vi "SeCrTS-DD NS Receiver Storage.vi"(8 "error in":errorcluster) -> ()   [LabVIEW 2022 SP3]
uses:
  Control/SeCrTS-Notifier Ref.ctl
  Globals/SeCrTS-DD globals.vi
  <resource>/objmgr/ni.dex.rc
panel:
  out "x":u32
  out "error out":errorcluster
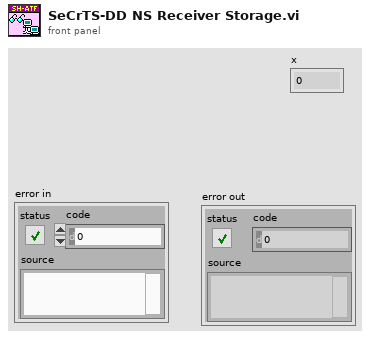
[diagram p1: front panel]
types:
  T1 = typedef "SeCrTS-Notifier Ref.ctl" = cluster{"Pump":refnum<notifier>, "Storage":refnum<notifier>}
  T2 = cluster{"In Progress":bool, "reader url":refnum<k21>, "DI P\nDI S":refnum<queue>[], "analog queue":refnum<queue>[], "NOT DIS Out":T1}
  T3 = enum16{"Initialize", "Wait for connection", "Send data", "Exit", "Receive Data"}
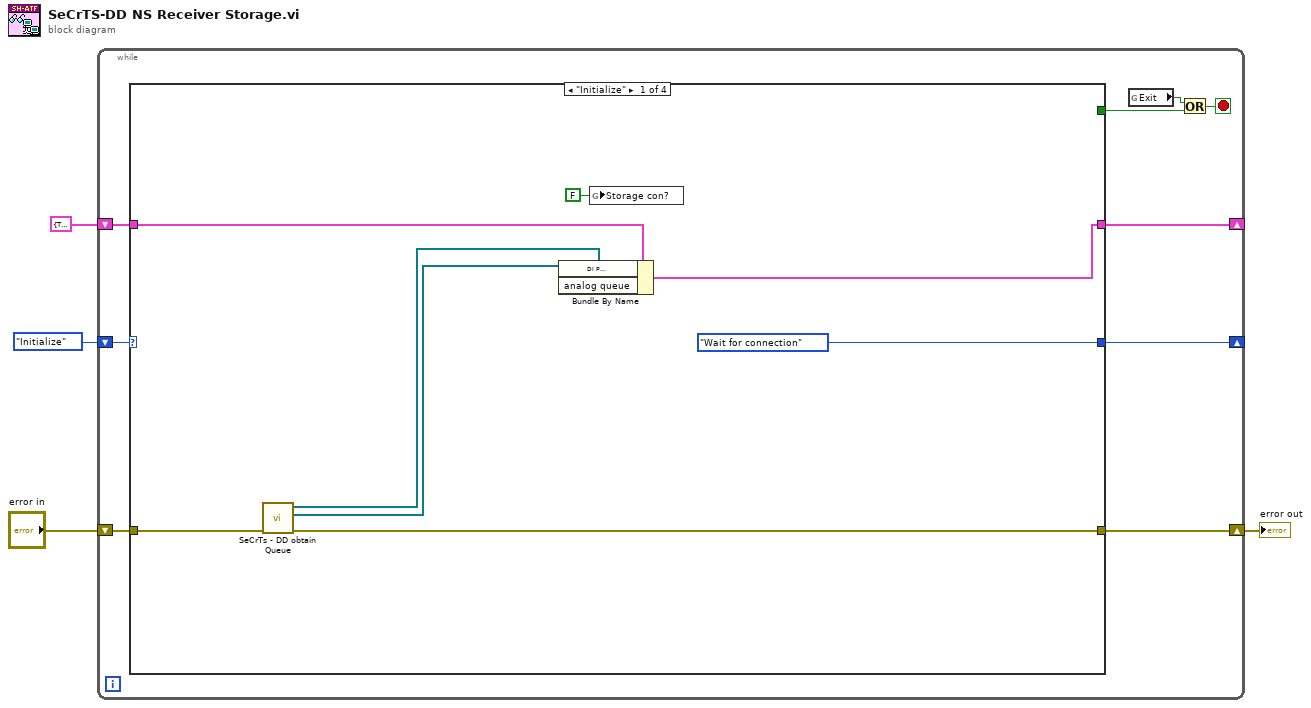
[diagram p0: block diagram]
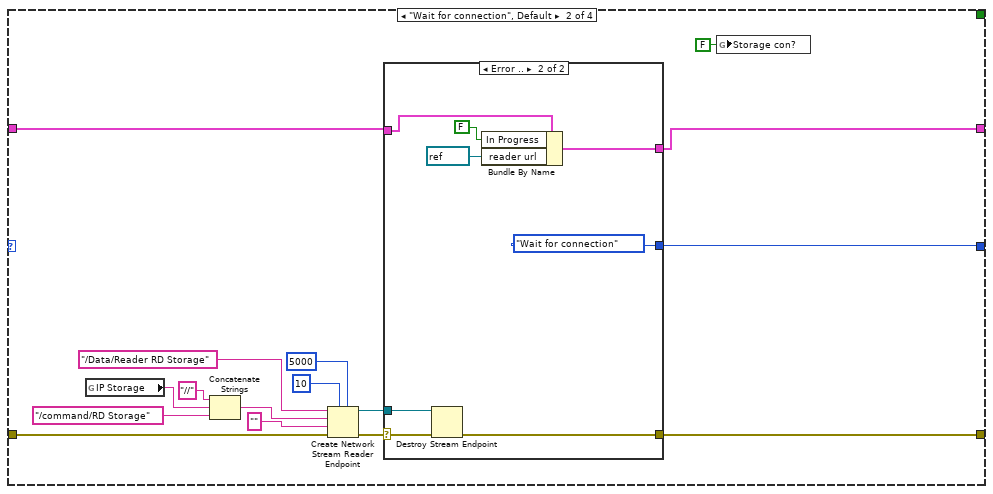
[diagram p2: hidden frame]
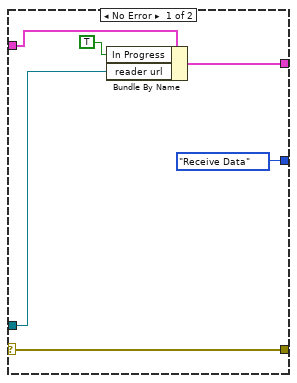
[diagram p3: hidden frame]
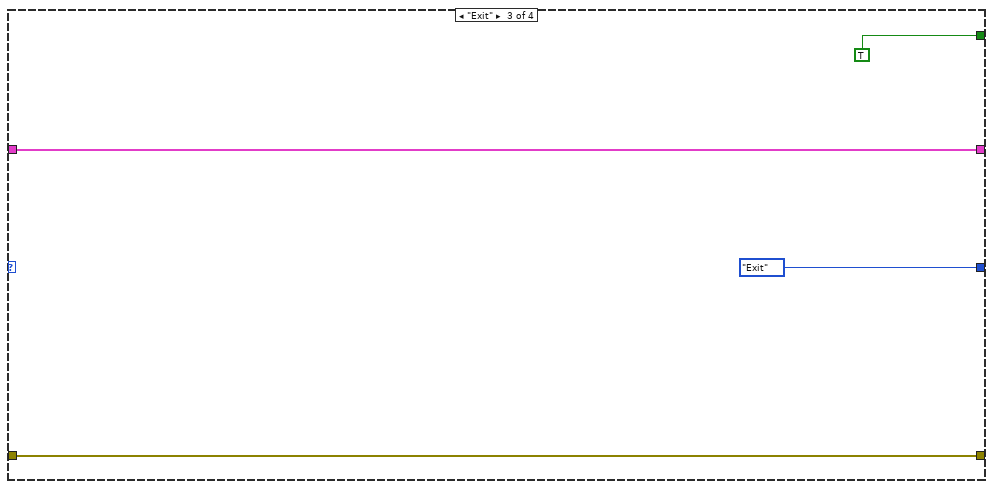
[diagram p4: hidden frame]
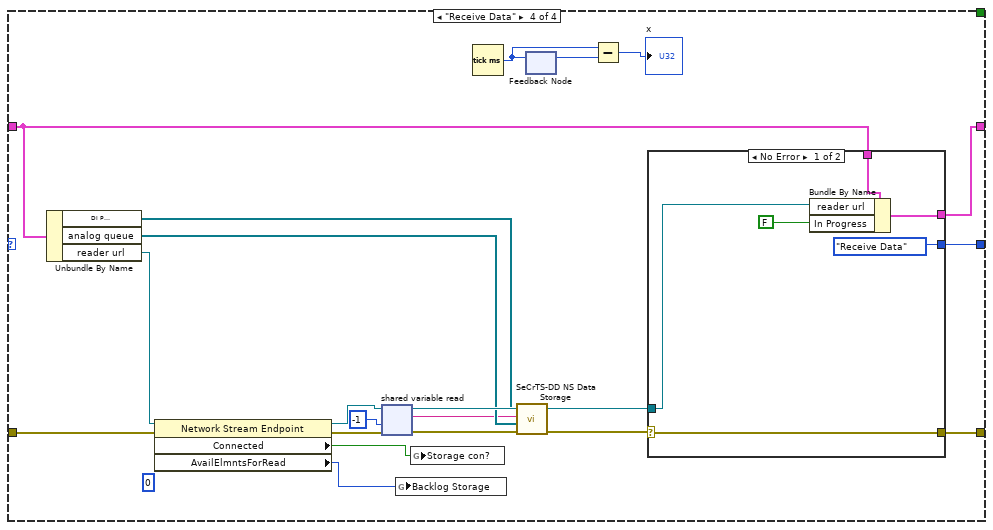
[diagram p5: hidden frame]
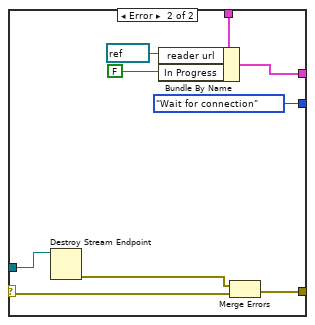
[diagram p6: hidden frame]
diagram:
  n1 = while {
    shift-right: [w11] -> _
    shift-left: T3."Initialize" -> [w13]
    shift-right: [w9] -> _
    shift-left: T2 {"In Progress"=TRUE, "reader url"="", "DI P\nDI S"=[], "analog queue"=[], "NOT DIS Out"={"Pump"=refnum, "Storage"=refnum}} -> [w10]
    shift-right: [w7] -> w2
    shift-left: "error in" -> [w8]
    stop <- w6 stop-if-true
    n2 = case shown="\"Initialize\"" w13 {
      tunnel: [_ _ TRUE _] -> w12
      tunnel: [T3."Wait for connection" w33 T3."Exit" w74] -> w11
      tunnel: w10 -> [w15 w37 w54 w57]
      tunnel: [w16 w36 w54 w58] -> w9
      tunnel: w8 -> [w20 w35 w52 w75]
      tunnel: [w19 w34 w52 w73] -> w7
      frame "Initialize" {
        n3 = call "SeCrTs - DD obtain Queue.vi"("error in"=w20) -> ("error out"=w19:errorcluster, "AI_V_Data P\nAI_C_Data P\nAO_Data P\nDO_Data P\nACC_Data P\nTC Data P\nDrive_A_C \nDrive_A_D\nAI_C_Data S\nDO_Data S\nAI_V_Rms_P"=w18:refnum<queue>[], "DI P\nDI S"=w17:refnum<queue>[])  [unwired: 8 in]
        n4 = Bundle By Name(cluster=w15, "DI P\nDI S"=w17, "analog queue"=w18) -> (w16:T2)
        n5 = global write "SeCrTS-DD globals.vi" "Storage con?"(FALSE ("Storage con?")) -> ()
      }
      frame "Wait for connection", Default {
        n6 = global read "SeCrTS-DD globals.vi" "IP Storage"() -> (w24:string)
        n7 = Concatenate Strings("//" ("string"), w24, "/command/RD Storage" ("reader url")) -> (w26:string)
        n8 = Create Network Stream Reader Endpoint(5:5000 ("timeout in ms (-1)"), 7:10 ("reader buffer size"), 8:w35, 9:"", 10:w26, 11:"/Data/Reader RD Storage" ("writer name")) -> (0:w30:errorcluster, 3:w31:refnum<k21>)  [unwired: 1 in]
        n9 = case shown="Error .." w30 {
          selector: w30 -> [w40 w47]
          tunnel: w37 -> [w43 w51]
          tunnel: w31 -> [w38 w48]
          tunnel: [w41 w50] -> w36
          tunnel: [w40 w46] -> w34
          tunnel: [T3."Receive Data" T3."Wait for connection"] -> w33
          frame No Error {
            n10 = Bundle By Name(cluster=w43, "In Progress"=TRUE, "reader url"=w38) -> (w41:T2)
          }
          frame Error {
            n11 = Destroy Stream Endpoint(8:w47, 11:w48) -> (0:w46:errorcluster)
            n12 = Bundle By Name(cluster=w51, "In Progress"=FALSE, "reader url"=refnum<k21> refnum) -> (w50:T2)
          }
        }
        n13 = global write "SeCrTS-DD globals.vi" "Storage con?"(FALSE ("Storage con?")) -> ()
      }
      frame "Exit" {
      }
      frame "Receive Data" {
        (unwired) 0 ("Available Elements for Reading")
        n14 = Unbundle By Name(w57) -> ("DI P\nDI S"=w62:refnum<queue>[], "analog queue"=w61:refnum<queue>[], "reader url"=w60:refnum<k21>)
        n15 = property class="Network Stream Endpoint"(reference=w60, error in=w75) -> (reference out=w72:refnum<k21>, error out=w71:errorcluster, "Connected"=w70:bool, "AvailElmntsForRead"=w56:i32)
        n16 = shared-variable-read(w72, w71, -1 ("timeout ms (-1)")) -> (w65:refnum<k21>, w64:errorcluster, w59:string)  [unwired: 1 out]
        n17 = global write "SeCrTS-DD globals.vi" "Backlog Storage"(w56) -> ()
        n18 = global write "SeCrTS-DD globals.vi" "Storage con?"(w70) -> ()
        n19 = Tick Count (ms)() -> (millisecond timer value=w68:u32)
        n20 = call "SeCrTS-DD NS Data Storage.vi"("error in"=w64, "AI_V_Data P\nAI_C_Data P\nAO_Data P\nDO_Data P\nACC_Data P\nTC Data P\nDrive_A_C \nDrive_A_D\nAI_C_Data S\nDO_Data S"=w61, "Data in"=w59, "DI P\nDI S"=w62) -> ("error out"=w63:errorcluster)  [unwired: 7 in]
        n21 = feedback #1() -> (w69:u32)  [unwired: 1 in]
        n22 = feedback-in #1(w68) -> ()
        n23 = Subtract(x=w68, y=w69) -> (x-y=→"x":u32)
        n24 = case shown="No Error" w63 {
          selector: w63 -> [w81 w82]
          tunnel: [w81 w84] -> w73
          tunnel: [T3."Receive Data" T3."Wait for connection"] -> w74
          tunnel: w65 -> [w76 w89]
          tunnel: w57 -> [w77 w88]
          tunnel: [w78 w86] -> w58
          frame No Error {
            n25 = Bundle By Name(cluster=w77, "reader url"=w76, "In Progress"=FALSE) -> (w78:T2)
          }
          frame Error {
            n26 = Destroy Stream Endpoint(11:w89) -> (0:w83:errorcluster)  [unwired: 1 in]
            n27 = Bundle By Name(cluster=w88, "reader url"=refnum<k21> refnum, "In Progress"=FALSE) -> (w86:T2)
            n28 = Merge Errors(w83, w82) -> (w84:errorcluster)
          }
        }
      }
    }
    n29 = global read "SeCrTS-DD globals.vi" "Exit"() -> (w5:bool)
    n30 = Or(x=w5, y=w12) -> (x .or. y?=w6:bool)
  }
  "error out" <- w2
